vi "Target.vi"() -> ()   [LabVIEW 2018]
uses:
  Statechart.lvsc/StatechartState.ctl
  Statechart.lvsc/State.ctl
  shared/Kobuki Sensor Display.ctl
  shared/Sensors.ctl
  shared/Accelerometer.ctl
  Kobuki/KobukiSensors.ctl
  Kobuki/Kobuki Bumps and WheelDrops.ctl
  Kobuki/Kobuki Buttons.ctl
  Statechart.lvsc/CompanionDiagram.vi/136/SC Main.vi
  Statechart.lvsc/CompanionDiagram.vi/136/Upd State.vi
  Statechart.lvsc/CompanionDiagram.vi/136/Trans Graph0.vi
  Statechart.lvsc/CompanionDiagram.vi/136/EnterGraphCore.vi
  <vilib>/myRIO/Common/Instrument Driver Framework/myRIO v1.0/UART/vis/myRIO v1.0 Close UART.vi
  Statechart.lvsc/CompanionDiagram.vi/136/Trans Graph1.vi
  Statechart.lvsc/CompanionDiagram.vi/136/Trans Graph2.vi
  <vilib>/myRIO/Common/Instrument Driver Framework/myRIO v1.0/myRIO v1.1 Open.vi
  Statechart.lvsc/CompanionDiagram.vi
  shared/Wrap Angle.vi
  <vilib>/myRIO/Common/Instrument Driver Framework/Utilities/vis/FPGA Ref Manager.vi
  <vilib>/myRIO/Common/Instrument Driver Framework/myRIO v1.0/myRIO v1.0 Reset FPGA.vi
  <vilib>/myRIO/Common/Instrument Driver Framework/myRIO v1.0/IRQ/vis/myRIO v1.0 IRQ Info FGV.vi
  <vilib>/myRIO/Common/Instrument Driver Framework/myRIO v1.0/IRQ/vis/myRIO v1.0 Timer IRQ Info FGV.vi
  <vilib>/myRIO/Common/Instrument Driver Framework/myRIO v1.0/IRQ/vis/myRIO v1.0 ISR Agent.vi
  Statechart.lvsc/Trigger.ctl
  <vilib>/Statechart/Infrastructure/RTStatechart/RunTime SCN.xnode
  Statechart.lvsc/Inputs.ctl
  Statechart.lvsc/Outputs.ctl
  Statechart.lvsc
  <vilib>/myRIO/Instrument Drivers/Utilities/Utilities.lvlib
panel:
  in  "Tab Control":T1(tab)
  out "Kobuki Sensors (graphical)":T2 {"Right Wheel (mm/s)" scale=-500.0..500.0; "Left Wheel (mm/s)" scale=-500.0..500.0}
  out "Active States":T4
  out "error out":errorcluster
  in  "stop":bool
  out "Target Running":bool
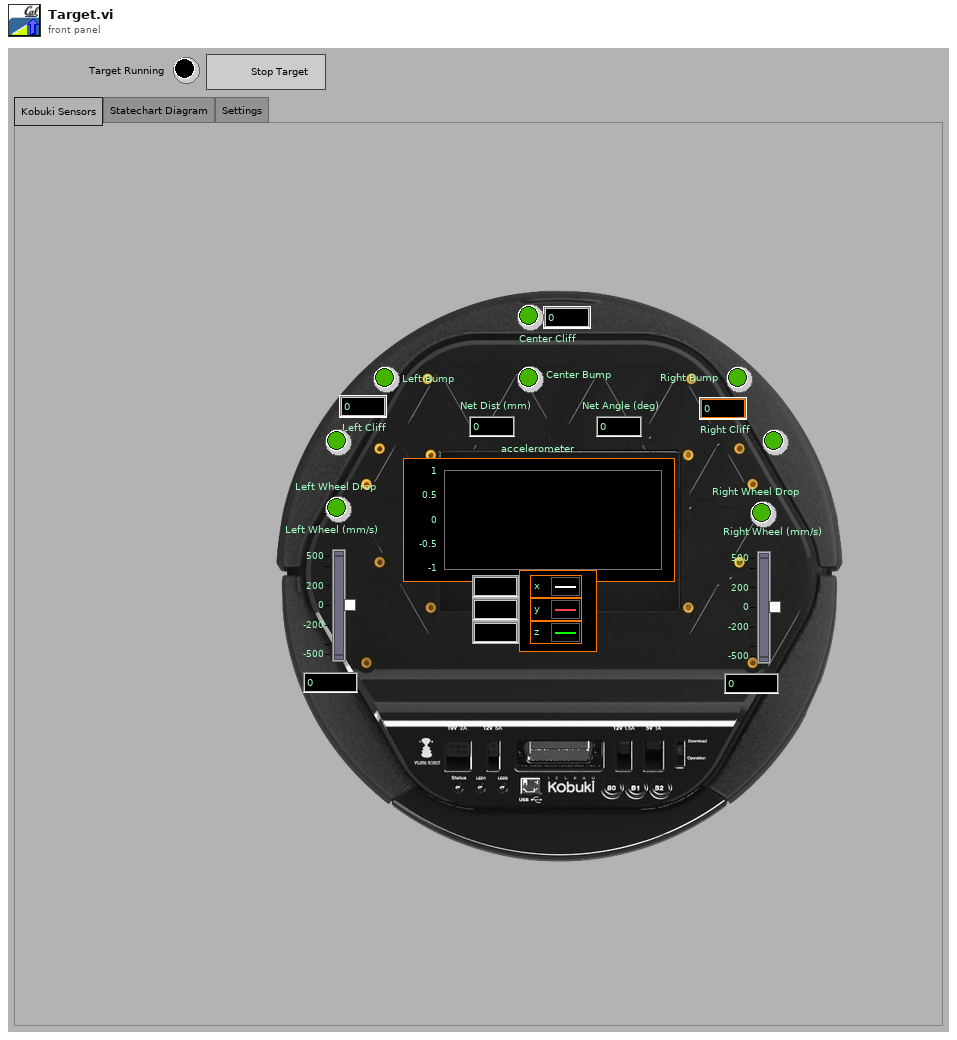
[diagram p1: front panel]
types:
  T1 = enum32{"Kobuki Sensors", "Statechart Diagram", "Settings"}
  T2 = typedef "Kobuki Sensor Display.ctl" = cluster{"Center Bump":bool, "Left Wheel Drop":bool, "Right Wheel Drop":bool, "Left Bump":bool, "Right Bump":bool, "Left Cliff":bool, "Center Cliff":bool, "Right Cliff":bool, "Net Dist (mm)":i32, "Net Angle (deg)":i32, "Left Cliff":u16, "Center Cliff":u16, "Right Cliff":u16, "  Left Wheel (mm/s)":i16, "Right Wheel (mm/s)":i16, "accelerometer":T3}
  T3 = typedef "Accelerometer.ctl" = cluster{"x axis (g)":dbl, "y axis (g)":dbl, "z axis (g)":dbl}
  T4 = typedef "Statechart.lvsc/StatechartState.ctl" = T5[]
  T5 = typedef "Statechart.lvsc/State.ctl" = enum16{"NI.SC.Initial", "NI.SC.History", "NI.SC.ShallowHistory", "NI.SC.Terminal", "Pause", "Run", "Pause\\Detect Play Button\\Pause;\nWait for\nbutton\nrelease", "Pause\\Detect Play Button\\Unpause;\nwait for\nbutton release", "Pause\\Detect Play Button\\Unpause;\nwait for\nbutton press", "Run\\Run Mode\\Initlialise", "Run\\Run Mode\\Stop", "Run\\Run Mode\\On Plateau", "Run\\Run Mode\\Sweep Right", "Run\\Run Mode\\Sweep Left", "Run\\Run Mode\\Drive Back from left", "Run\\Run Mode\\Drive Back from right", "Run\\Run Mode\\Orient Hill", "Run\\Run Mode\\Drive Hill", "Run\\Run Mode\\Reorient from L", "Run\\Run Mode\\Reorient from R", "Run\\Run Mode\\Drive Forward from R", "Run\\Run Mode\\Drive Forward from L", "Run\\Run Mode\\Turn Right ", "Run\\Run Mode\\Turn Left", "Run\\Run Mode\\Drive"}
  T6 = typedef "Sensors.ctl" = cluster{"net distance (mm)":i32, "net angle (deg)":i32, "accelerometer":T3, "Is Simulator?":bool, "Kobuki Sensors":T7, "Requested Left Wheel Velocity(mm/s)":i32, "Requested Right Wheel Velocity(mm/s)":i32}
  T7 = typedef "KobukiSensors.ctl" = cluster{"Bumps + Wheel Drops":T8, "Cliff Left":bool, "Cliff Center":bool, "Cliff Right":bool, "Cliff Left Signal":u16, "Cliff Center Signal":u16, "Cliff Right Signal":u16, "Buttons":T9, "Left Wheel Encoder (ticks)":u16, "Right Wheel Encoder (ticks) ":u16, "Left  Wheel PWM":i8, "Right Wheel PWM":i8, "Left Wheel OverCurrent":bool, "Right Wheel OverCurrent ":bool, "Right Wheel Current (x10mA)":i16, "Left  Wheel Current  (x10mA)":i16, "TimeStamp":u16, "Battery Voltage (mV)":i16, "Angle( of 100deg)":i16, "Angle Rate( of 100 deg/sec)":i16, "Charger Source ":i8}
  T8 = typedef "Kobuki Bumps and WheelDrops.ctl" = cluster{"Wheeldrop Left":bool, "Wheeldrop Right":bool, "Bump Left":bool, "Bump Center":bool, "Bump Right":bool}
  T9 = typedef "Kobuki Buttons.ctl" = cluster{"B0":bool, "B1":bool, "B2":bool}
  T10 = typedef "Statechart.lvsc/Outputs.ctl" = cluster{"Left Wheel Speed (mm/s)":i16, "Right Wheel Speed (mm/s)":i16, "onHill":i16, "hillAngle":i16, "reachedPlateau":i16, "onHillThreshold":i16, "orientateXThreshold":i16, "orientateYThreshold":i16}
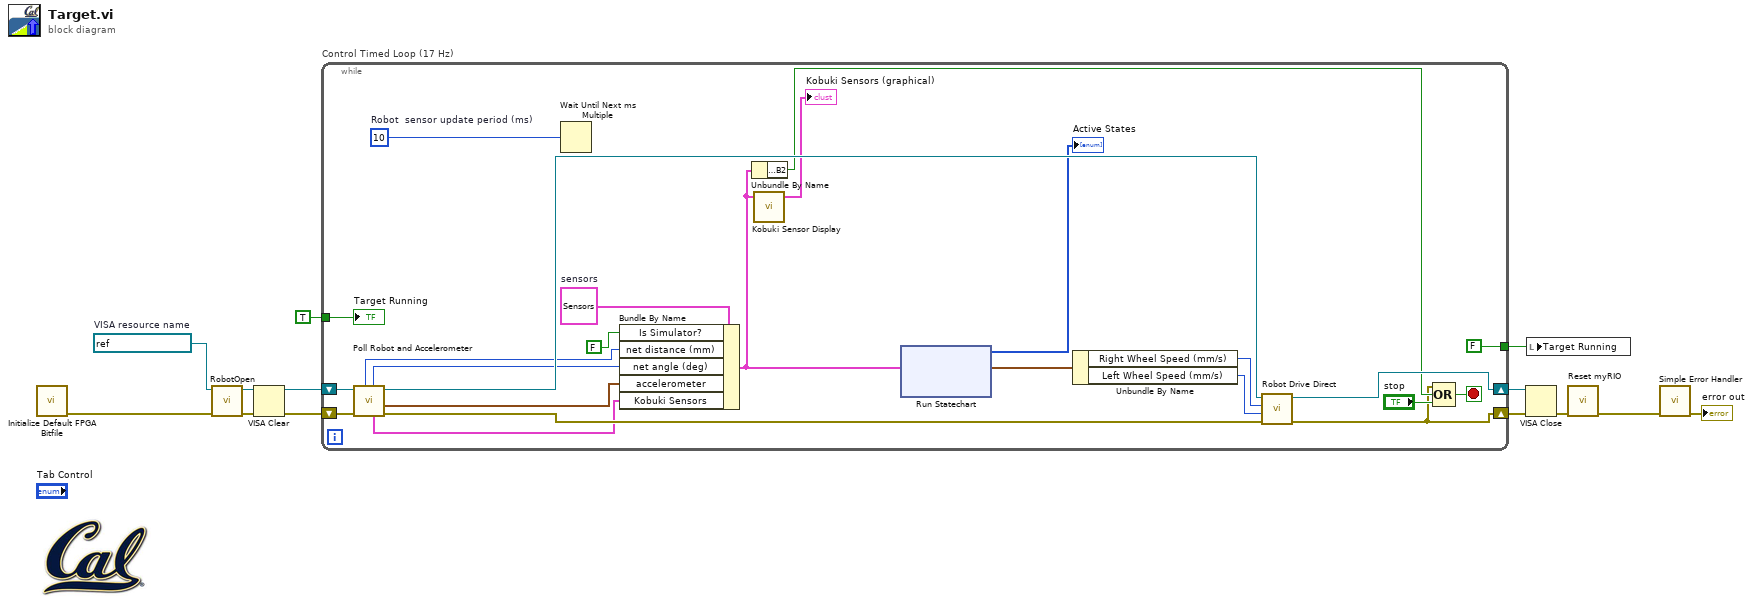
[diagram p0: block diagram]
diagram:
  w10 = refnum<visa-resource-name> "ASRL2::INSTR"  # VISA resource name
  n1 = call <vilib>:"Initialize Default FPGA Bitfile.vi"() -> ("error out"=w8:errorcluster)  [unwired: 11 in]
  n2 = call "RobotOpen.vi"("error in (no error)"=w8, "Robot Communication port name"=w10) -> ("error out"=w6:errorcluster, "Robot Communication port name out"=w13:refnum<visa-resource-name>)  [unwired: 8 in]
  n3 = VISA Clear(VISA resource name=w13, error in (no error)=w6) -> (VISA resource name out=w4:refnum<visa-resource-name>, error out=w5:errorcluster)
  n4 = while "Control Timed Loop (17 Hz)" {
    shift-right: [w37] -> w2
    shift-left: w4 -> [w33]
    shift-right: [w19] -> w3
    shift-left: w5 -> [w32]
    tunnel: TRUE ("stop") -> [w27]
    tunnel: [FALSE ("stop")] -> w11
    stop <- w36 stop-if-true
    w20 = T6 {"net distance (mm)"=0, "net angle (deg)"=0, "accelerometer"={"x axis (g)"=0.0, "y axis (g)"=0.0, "z axis (g)"=0.0}, "Is Simulator?"=FALSE, "Kobuki Sensors"={"Bumps + Wheel Drops"={"Wheeldrop Left"=FALSE, "Wheeldrop Right"=FALSE, "Bump Left"=FALSE, "Bump Center"=FALSE, "Bump Right"=FALSE}, "Cliff Left"=FALSE, "Cliff Center"=FALSE, "Cliff Right"=FALSE, "Cliff Left Signal"=0, "Cliff Center Signal"=0, "Cliff Right Signal"=0, "Buttons"={"B0"=FALSE, "B1"=FALSE, "B2"=FALSE}, "Left Wheel Encoder (ticks)"=0, "Right Wheel Encoder (ticks) "=0, "Left  Wheel PWM"=0, "Right Wheel PWM"=0, "Left Wheel OverCurrent"=FALSE, "Right Wheel OverCurrent "=FALSE, "Right Wheel Current (x10mA)"=0, "Left  Wheel Current  (x10mA)"=0, "TimeStamp"=0, "Battery Voltage (mV)"=0, "Angle( of 100deg)"=0, "Angle Rate( of 100 deg/sec)"=0, "Charger Source "=0}, "Requested Left Wheel Velocity(mm/s)"=0, "Requested Right Wheel Velocity(mm/s)"=0}  # sensors
    w22 = u32 10  # Robot  sensor update period (ms)
    n5 = call "Poll Robot and Accelerometer.vi"("error in"=w32, "UART in"=w33) -> ("error out"=w31:errorcluster, "Acceleration (g)"=w23:T3, "UART out"=w30:refnum<visa-resource-name>, "Kobuki Sensors  out"=w16:T7, "net angle (deg)"=w28:i32, "net distance (mm)"=w29:i32)  [unwired: 4 in]
    n6 = Wait Until Next ms Multiple(millisecond multiple=w22) -> ()  [unwired: 1 out]
    n7 = Bundle By Name(cluster=w20, "Is Simulator?"=FALSE, "net distance (mm)"=w29, "net angle (deg)"=w28, "accelerometer"=w23, "Kobuki Sensors"=w16) -> (w14:T6)
    n8 = Unbundle By Name(w14) -> ("Kobuki Sensors.Buttons.B2"=w24:bool)
    n9 = call "Kobuki Sensor Display.vi"("sensors"=w14) -> ("Kobuki Sensors Display"=→"Kobuki Sensors (graphical)":T2)  [unwired: 4 in]
    n10 = xnode "Run Statechart"("Inputs"=w14) -> ("Outputs"=w35:T10, "Active States"=→"Active States":T4)  [unwired: 2 in, 1 out]
    n11 = Unbundle By Name(w35) -> ("Right Wheel Speed (mm/s)"=w18:i16, "Left Wheel Speed (mm/s)"=w17:i16)
    n12 = call "Robot Drive Direct.vi"("error in"=w31, "Left Wheel Velocity (mm/s)"=w17, "Right Wheel Velocity (mm/s)"=w18, "UART port in"=w30) -> ("error out"=w19:errorcluster, "UART port out"=w37:refnum<visa-resource-name>)  [unwired: 6 in]
    n13 = Compound Arithmetic op=OR(w19, w24, "stop") -> (w36:bool)
    "Target Running" <- w27
  }
  n14 = VISA Close(VISA resource name=w2, error in (no error)=w3) -> (error out=w1:errorcluster)
  n15 = local write "Target Running"(w11) -> ()
  n16 = call <vilib>:"Reset myRIO.vi"("error in (no error)"=w1) -> ("error out"=w9:errorcluster)  [unwired: 10 in]
  n17 = call <vilib>:"Simple Error Handler.vi"("error in (no error)"=w9) -> ("error out"=→"error out":errorcluster)  [unwired: 4 in, 4 out]
